vi "Part-2.vi"() -> ()   [LabVIEW 2015]
panel:
  out "Complex Arrays":cdb[][](array[numeric])
  out "x+y":cdb[](array[numeric])
  in  "w":cdb[](array[numeric])
  out "Imaginary":dbl[](array[numeric])
  out "Real":dbl[](array[numeric])
  out "Theta":dbl[](array[numeric])
  out "Magnitude":dbl[](array[numeric])
  in  "z":cdb[](array[numeric])
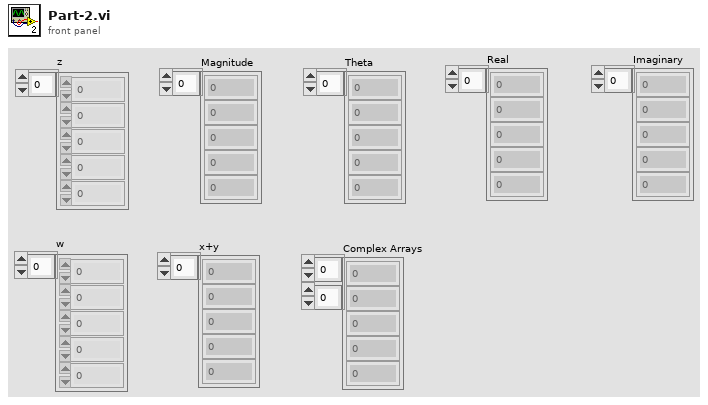
[diagram p1: front panel]
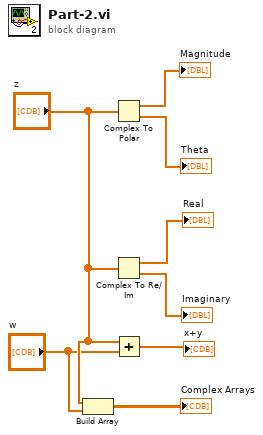
[diagram p0: block diagram]
diagram:
  n1 = Build Array("z", "w") -> (→"Complex Arrays":cdb[][])
  n2 = Complex To Polar(r * e^(i*theta)="z") -> (r=→"Magnitude":dbl[], theta=→"Theta":dbl[])
  n3 = Complex To Re/Im(x + iy="z") -> (x=→"Real":dbl[], y=→"Imaginary":dbl[])
  n4 = Add(x="z", y="w") -> (x+y=→"x+y":cdb[])
